vi "LVObject to JSON - Error in To JSON - Returns Empty String.vi"() -> ()   [LabVIEW 2017, in "JSON Serializable Serializer Tests.lvlib"]
uses:
  JSON Serializable Serializer Tests.lvlib
  JSON Serializable Serializer/JSON Serializable Serializer.lvclass
  <vilib>/Utility/error.llb/Error Cluster From Error Code.vi
  <vilib>/addons/_JKI Toolkits/Caraya/classes/Assert/Assert Equal Value_Variant.vi
  <vilib>/ErrorRing/Error Ring.xnode
  <vilib>/addons/_JKI Toolkits/Caraya/classes/Test/Test.lvclass
  <vilib>/addons/_JKI Toolkits/Caraya/classes/Assert/Assert.lvclass
  Mock JSON Serializable/Mock JSON Serializable.lvclass
panel:
  out "error out":errorcluster
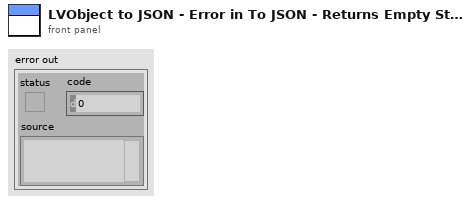
[diagram p1: front panel]
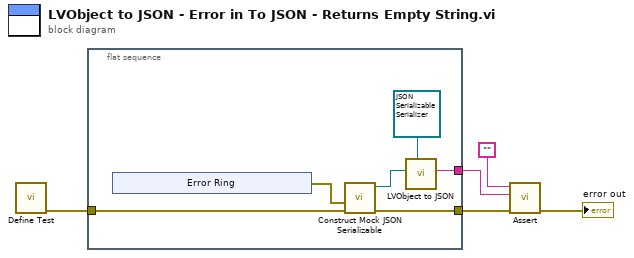
[diagram p0: block diagram]
diagram:
  n1 = call <vilib>:"Define Test.vi"() -> ("error out"=w4:errorcluster)  [unwired: 11 in]
  n2 = flat-sequence {
    tunnel: [w10] -> w5
    tunnel: w4 -> [w9]
    tunnel: [w6] -> w2
    frame #0 {
      n3 = xnode "Error Ring"() -> ("error out"=w7:errorcluster)
      n4 = call "Construct Mock JSON Serializable.vi"("error in (no error)"=w9, "From/To JSON <error out> (no error)"=w7) -> ("error out"=w10:errorcluster, "Mock JSON Serializable"=w8:refnum<class "Mock JSON Serializable.lvclass">)  [unwired: 8 in]
      n5 = call-dynamic "LVObject to JSON.vi"("JSON Serializer in"=refnum<class "JSON Serializable Serializer.lvclass"> refnum ("JSON Serializer.lvclass"), "Object"=w8) -> ("<JSON>Object"=w6:string)  [unwired: 8 in, 1 out]
    }
  }
  n6 = call-poly <vilib>:"Assert.vi"("error in (no error)"=w5, "Y"=w2, "X"="") -> ("error out"=→"error out":errorcluster)  [unwired: 8 in]
